vi "CAN_ReadBMS.vi"(8 "error in (no error)":errorcluster) -> (0 "error out":errorcluster)   [LabVIEW 2018]
uses:
  BMS/OrionBMSClass.lvclass
  <vilib>/Platform/TimedLoop/XDataNode/timing_clust.ctl
  <vilib>/Platform/TimedLoop/XDataNode/nitl_modes.ctl
  <vilib>/Platform/TimedLoop/XDataNode/wakeup.ctl
  Type_Def/Type_Def Actuator Controls.ctl
  Type_Def/TypeDef_BMSDatas.ctl
  Type_Def/TypeDef_BMSStatuss.ctl
  <vilib>/Platform/TimedLoop/XDataNode/XDataNode.xnode
  <vilib>/Platform/TimedLoop/XDataNode/XDNodeRunTimeDep.lvlib
panel:
  out "DeviceFroze":bool=TRUE
  out "Loop Counter":i32
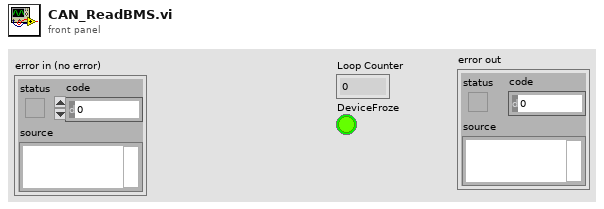
[diagram p1: front panel]
types:
  T1 = enum32{"1 Mbit/s", "800 kbit/s", "500 kbit/s", "250 kbit/s", "125 kbit/s", "50 kbit/s", "20 kbit/s", "10 kbit/s", ""}
  T2 = typedef "XDNodeRunTimeDep.lvlib/timing_clust.ctl" = cluster{"Expected End [f-1]":u64, "Actual End [f-1]":u64, "Finished Late? [f-1]":bool, "Expected End [i-1]":u64, "Actual End [i-1]":u64, "Finished Late? [i-1]":bool, "Expected Start [i]":u64, "Actual Start [i]":u64, "Expected Start [f]":u64, "Actual Start [f]":u64, "Source Name":string, "Structure Name":string, "Period":i64, "Deadline":i64, "Offset":i64, "Start":i64, "Priority":i32, "Timeout":i32, "Mode":T3, "Wakeup Reason":T4, "Error":errorcluster, "Source Type":string, "Secondary Source Type":string, "Global End Time":u64, "Global Start Time":u64, "Frame Duration":u64, "Iteration Duration":u64, "Assigned CPU":i32, "I/O Scan Engine Mode":u32}
  T3 = typedef "XDNodeRunTimeDep.lvlib/nitl_modes.ctl" = enum32{"No Change", "Process missed periods, maintain original phase", "Discard missed periods, maintain original phase", "Process missed periods, ignore original phase", "Discard missed periods, ignore original phase"}
  T4 = typedef "XDNodeRunTimeDep.lvlib/wakeup.ctl" = enum32{"Normal", "Aborted", "Asynchronous wakeup", "Timing source error", "Timed loop error", "Timeout"}
  T5 = typedef "Type_Def Actuator Controls.ctl" = cluster{"Reverse ":bool, "Precharge Ctrl":bool, "Pump Ctrl":bool, "24 VDC Ctr":bool, "Vent Solenoid":bool, "Brake Solenoid":bool, "EMCY  Brake Solenoid":bool, "Digital Out 7B ":bool, "Forward Ctrl":bool, "Contact H1":bool, "Contact L1":bool, "Contact H2":bool, "Contact L2 ":bool, "LED RED":bool, "LED GREEN":bool, " Digital Out 7A":bool}
  T6 = typedef "TypeDef_BMSDatas.ctl" = cluster{"Pack 1 Max Cell\n Voltage (V)":dbl, "Pack 1 Max Cell\n ID ":dbl, "Pack 1 Min Cell \nVoltage (V)":dbl, "Pack 1 Min Cell \nID ":dbl, "Pack 1 State of Charge  (%)":dbl, "Pack 1 Average Voltage1 (V)":dbl, "Pack 1Voltage Delta (V)":dbl, "Pack 1 Current (A)":dbl, "Pack 1 Voltage (V)":dbl, "Pack 1 Max Resistance (Ohm)":dbl, "Pack 1Min Resistance (Ohm)":dbl, "Pack 1Average Resistance (Ohm)":dbl, "Pack 1Delta Resistance (Ohm)":dbl, "Pack 1 Highest Temperature(F)":dbl, "BmsStatus":T7, "Pack 2 Max Cell\n Voltage (V) ":dbl, "Pack 2 Max Cell\n ID  ":dbl, "Pack 2 Min Cell \nVoltage (V) ":dbl, "Pack 2 Min Cell \nID  ":dbl, "Pack 2 Average Voltage1 (V)":dbl, "Pack 2 Voltage Delta (V) ":dbl, "Pack 2 Current (A)":dbl, "Pack 2 Voltage (V) ":dbl, "Pack 2 State of Charge  (%) ":dbl, "Pack 2 Max Resistance (Ohm) ":dbl, "Pack 2 Min Resistance (Ohm)":dbl, "Pack 2 Average Resistance (Ohm)":dbl, "Pack 2 Delta Resistance (Ohm) ":dbl, "Pack 2 Highest Temperature(F) ":dbl}
  T7 = typedef "TypeDef_BMSStatuss.ctl" = cluster{"isFault":bool, "isolationMonitoring":bool, "isFault 2":bool, "isolationMonitoring 2":bool}
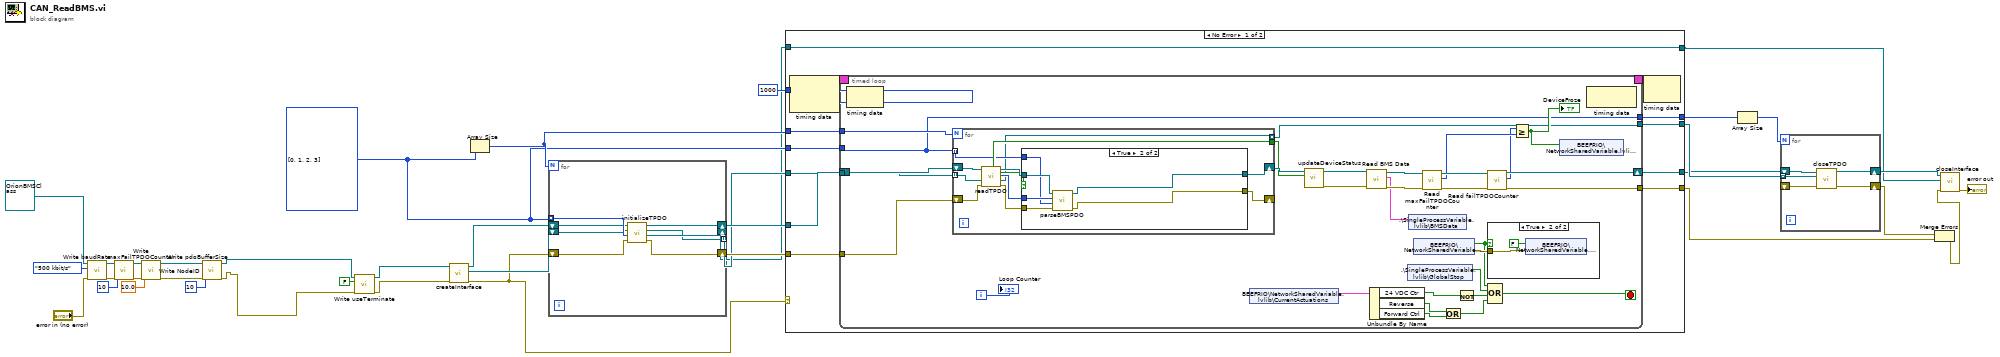
[diagram p0: block diagram]
diagram:
  w26 = u8[] [0, 1, 2, 3] items=["PDO 1", "PDO 2", "PDO 3", "PDO 4"]
  n1 = call-dynamic "Write baudRate.vi"("error in (no error)"="error in (no error)", "baudRate"=T1."500 kbit/s", "OrionBMSClass in"=refnum<class "OrionBMSClass.lvclass"> refnum ("OrionBMSClass.lvclass")) -> ("error out"=w13:errorcluster, "OrionBMSClass out"=w7:refnum<class "OrionBMSClass.lvclass">)  [unwired: 7 in]
  n2 = call-dynamic "Write maxFailTPDOCounter.vi"("error in (no error)"=w13, "maxFailTPDOCounter"=u8 10, "OrionBMSClass in"=w7) -> ("error out"=w12:errorcluster, "OrionBMSClass out"=w8:refnum<class "OrionBMSClass.lvclass">)  [unwired: 7 in]
  n3 = call-dynamic "Write NodeID.vi"("error in (no error)"=w12, "NodeID"=10.0, "OrionBMSClass in"=w8) -> ("error out"=w14:errorcluster, "OrionBMSClass out"=w9:refnum<class "OrionBMSClass.lvclass">)  [unwired: 7 in]
  n4 = call-dynamic "Write pdoBufferSize.vi"("error in (no error)"=w14, "pdoBufferSize"=u16 10, "OrionBMSClass in"=w9) -> ("error out"=w11:errorcluster, "OrionBMSClass out"=w10:refnum<class "OrionBMSClass.lvclass">)  [unwired: 7 in]
  n5 = call-dynamic "Write useTerminate .vi"("error in (no error)"=w11, "useTerminate"=FALSE, "OrionBMS in"=w10) -> ("error out"=w36:errorcluster, "OrionBMS out"=w33:refnum<class "OrionBMSClass.lvclass">)  [unwired: 7 in]
  n6 = call "createInterface.vi"("error in (no error)"=w36, "OrionBMS in"=w33) -> ("error out"=w31:errorcluster, "interface object out"=w34:refnum<k20>, "OrionBMS out"=w35:refnum<class "OrionBMSClass.lvclass">)  [unwired: 7 in]
  n7 = Array Size(array=w26) -> (size(s)=w30:i32)
  n8 = for {
    N: w30 -> [_]
    tunnel: w26 -> [w45] mode=indexing
    shift-right: [w39] -> w28
    shift-left: w31 -> [w42]
    shift-right: [w40] -> w21
    shift-left: w34 -> [w43]
    shift-right: [w41] -> w29
    shift-left: w35 -> [w44]
    tunnel: [w38] -> w27 mode=indexing
    n9 = call "initializeTPDO.vi"("error in (no error)"=w42, "PDO channel"=w45, "interface object in"=w43, "OrionBMS in"=w44) -> ("error out"=w39:errorcluster, "interface object out"=w40:refnum<k20>, "TPDO object out"=w38:refnum<k20>, "OrionBMS out"=w41:refnum<class "OrionBMSClass.lvclass">)  [unwired: 2 in]
  }
  n10 = case shown="No Error" w31 {
    tunnel: i64 1000 ("Period") -> [w56 _]
    tunnel: w30 -> [w55 _]
    tunnel: w29 -> [w54 w118]
    tunnel: w28 -> [w51 w117]
    tunnel: w27 -> [w53 w119]
    tunnel: w26 -> [w52 w120]
    tunnel: [w50 w120] -> w25
    tunnel: [w49 w119] -> w23
    tunnel: [w48 w118] -> w22
    tunnel: [w47 w117] -> w18
    tunnel: w21 -> [w46 w121]
    tunnel: [w46 w121] -> w16
    frame No Error {
      n11 = node-c288(w56) -> (w58:T2)  [unwired: 1 in]
      n12 = timed-loop {
        timing: w58 -> [_]
        timing-out: [_] -> w57
        tunnel: w55 -> [w86]
        shift-right: [w79] -> w48
        shift-left: w54 -> [w88]
        tunnel: w53 -> [w87]
        tunnel: w52 -> [w69]
        tunnel: [w72] -> w47
        tunnel: w51 -> [w71]
        tunnel: [w70] -> w49
        tunnel: [w69] -> w50
        i -> [w89]
        stop <- w62 stop-if-true
        n13 = node-c288() -> ()  [unwired: 1 in, 1 out]
        n14 = for {
          N: w86 -> [_]
          shift-right: [w95] -> w85
          shift-left: w88 -> [w102]
          tunnel: w87 -> [w98] mode=indexing
          tunnel: [w97] -> w84
          tunnel: w69 -> [w96] mode=indexing
          tunnel: [w94] -> w70 mode=indexing
          shift-right: [w92] -> _
          shift-left: w71 -> [w93]
          n15 = call "readTPDO.vi"("OrionBMS.lvclass"=w102, "TPDO object in"=w98, "error in (no error)"=w93) -> ("new data?"=w97:bool, "OrionBMS.lvclass"=w99:refnum<class "OrionBMSClass.lvclass">, "TPDO data"=w101:u8[], "TPDO object out"=w94:refnum<k20>, "error out"=w100:errorcluster)  [unwired: 3 in]
          n16 = case shown="True" w97 {
            tunnel: w101 -> [_ w110]
            tunnel: w100 -> [w103 w109]
            tunnel: w99 -> [w104 w108]
            tunnel: w96 -> [_ w107]
            tunnel: [w103 w105] -> w92
            tunnel: [w104 w106] -> w95
            frame False {
            }
            frame True {
              n17 = call "parseBMSPDO.vi"("error in (no error)"=w109, "PDO channel"=w107, "TPDO data"=w110, "OrionBMS in"=w108) -> ("error out"=w105:errorcluster, "OrionBMS out"=w106:refnum<class "OrionBMSClass.lvclass">)  [unwired: 6 in]
            }
          }
        }
        n18 = shared-variable "BEEFRIO\\NetworkSharedVariable.lvlib\\CurrentActuations"() -> (w68:T5)  [unwired: 1 in, 1 out]
        n19 = call "updateDeviceStatus.vi"("OrionBMS in"=w85, "isNewData"=w84) -> ("OrionBMS out"=w83:refnum<class "OrionBMSClass.lvclass">, "error out"=w82:errorcluster)  [unwired: 7 in]
        n20 = call-dynamic "Read BMS Data.vi"("error in (no error)"=w82, "OrionBMS in"=w83) -> ("error out"=w78:errorcluster, "BMS Data"=w76:T6, "OrionBMS out"=w81:refnum<class "OrionBMSClass.lvclass">)  [unwired: 7 in]
        n21 = Unbundle By Name(w68) -> ("24 VDC Ctr"=w67:bool, "Reverse"=w61:bool, "Forward Ctrl"=w60:bool)
        n22 = shared-variable ".\\SingleProcessVariable.lvlib\\GlobalStop"() -> (w65:bool)  [unwired: 1 in, 1 out]
        n23 = shared-variable ".\\SingleProcessVariable.lvlib\\BMSData"(w76) -> ()  [unwired: 1 in, 1 out]
        n24 = shared-variable "BEEFRIO\\NetworkSharedVariable.lvlib\\ReintCAN"() -> (w63:bool, error out=w64:errorcluster)  [unwired: 1 in]
        n25 = call-dynamic "Read maxFailTPDOCounter.vi"("error in (no error)"=w78, "OrionBMS in"=w81) -> ("error out"=w77:errorcluster, "maxFailTPDOCounter"=w75:u8, "OrionBMS out"=w80:refnum<class "OrionBMSClass.lvclass">)  [unwired: 7 in]
        n26 = Or(x=w61, y=w60) -> (x .or. y?=w59:bool)
        n27 = Not(x=w67) -> (.not. x?=w66:bool)
        n28 = call-dynamic "Read failTPDOCounter.vi"("error in (no error)"=w77, "OrionBMS in"=w80) -> ("error out"=w72:errorcluster, "failTPDOCounter"=w74:u8, "OrionBMS out"=w79:refnum<class "OrionBMSClass.lvclass">)  [unwired: 7 in]
        n29 = case shown="True" w63 {
          tunnel: w64 -> [_ w91]
          frame False {
          }
          frame True {
            n30 = shared-variable "BEEFRIO\\NetworkSharedVariable.lvlib\\ReintCAN"(FALSE ("ReintCAN"), error in=w91) -> ()  [unwired: 1 out]
          }
        }
        n31 = Compound Arithmetic op=OR(w63, w65, w66, w59) -> (w62:bool)
        n32 = Greater Or Equal?(x=w74, y=w75) -> (x >= y?=w73:bool)
        "DeviceFroze" <- w73
        n33 = shared-variable "BEEFRIO\\NetworkSharedVariable.lvlib\\BMSFreeze"(w73) -> ()  [unwired: 1 in, 1 out]
        n34 = node-c288() -> ()  [unwired: 1 in, 1 out]
        "Loop Counter" <- w89
      }
      n35 = node-c288(w57) -> ()  [unwired: 1 out]
    }
    frame Error {
    }
  }
  n36 = Array Size(array=w25) -> (size(s)=w24:i32)
  n37 = for {
    N: w24 -> [_]
    tunnel: w23 -> [w126] mode=indexing
    shift-right: [w123] -> w19
    shift-left: _ -> [w124]
    shift-right: [w122] -> w20
    shift-left: w22 -> [w125]
    n38 = call "closeTPDO.vi"("error in (no error)"=w124, "TPDO object in"=w126, "OrionBMSClass in"=w125) -> ("error in (no error) 2"=w123:errorcluster, "OrionBMSClass out"=w122:refnum<class "OrionBMSClass.lvclass">)  [unwired: 7 in]
  }
  n39 = Merge Errors(w19, w18) -> (w17:errorcluster)
  n40 = call "closeInterface.vi"("error in (no error)"=w17, "interface object in"=w16, "OrionBMS.lvclass"=w20) -> ("error out"=→"error out":errorcluster)  [unwired: 5 in, 1 out]
